vi "CheckState.vi"(8 "Error In":errorcluster, 10 "With sound?":bool, 11 "Astromech droid in":refnum<class "Astromech droid.lvclass">) -> (0 "Error Out":errorcluster, 3 "Astromech droid out":refnum<class "Astromech droid.lvclass">)   [LabVIEW 2021, in "Astromech droid.lvclass"]
uses:
  Astromech droid.lvclass
  Astromech droid.lvclass/Astromech droid.ctl
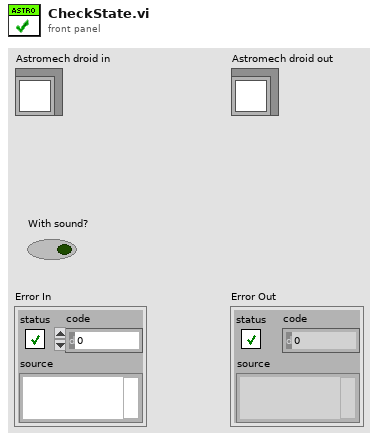
[diagram p1: front panel]
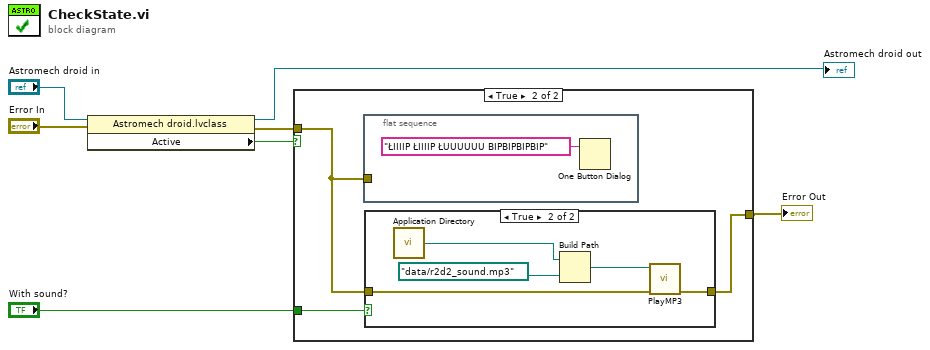
[diagram p0: block diagram]
diagram:
  n1 = property class="Astromech droid.lvclass"(reference="Astromech droid in", error in="Error In") -> (reference out=→"Astromech droid out":refnum<class "Astromech droid.lvclass">, error out=w6:errorcluster, "Active"=w7:bool)
  n2 = case shown="True" w7 {
    tunnel: [w8 w11] -> w3
    tunnel: "With sound?" -> [_ w9]
    tunnel: w6 -> [w8 w10]
    frame False {
    }
    frame True {
      n3 = flat-sequence {
        tunnel: w10 -> [_]
        frame #0 {
          n4 = One Button Dialog(message="ŁIIIIP ŁIIIIP ŁUUUUUU BIPBIPBIPBIP") -> ()  [unwired: 1 in, 1 out]
        }
      }
      n5 = case shown="True" w9 {
        tunnel: w10 -> [w13 w15]
        tunnel: [w13 w14] -> w11
        frame False {
        }
        frame True {
          n6 = call <vilib>:"Application Directory.vi"() -> ("Application Directory"=w16:path)
          n7 = Build Path(base path=w16, name or relative path=path "data/r2d2_sound.mp3") -> (appended path=w18:path)
          n8 = call "PlayMP3.vi"("Error In"=w15, "Path"=w18) -> ("Error out"=w14:errorcluster)  [unwired: 9 in]
        }
      }
    }
  }
  "Error Out" <- w3
